vi "PatternMatch_MainFunction.vi"(0 "PatternMatchParameter":T5={"Algorithm"=2, "Match Parameters"={"Number of Matches Requested"=1, "Minimum Match Score"=750.0, "Angle Ranges"=[]}, "ROI Descriptor"={"Global Rectangle"=[], "Contours"=[]}, "Advanced Options"=[{"Item"=1, "Value"=1.0}, {"Item"=103, "Value"=1.0}], "Template path"="", "XOffset"=0, "YOffset"=0} {"ROI Descriptor"."Contours"."Type" items=["No Selection", "Point", "Line", "Rectangle", "Oval", "Polygon", "Freehand Region", "Annulus", "Unused2", "Unused3", "Broken Line", "Freehand Line", "Rotated Rectangle"]; "Advanced Options"."Item" items=["LD Sampling - Minimum Constrast"=0, "LD Sampling - Enable Subpixel Accuracy"=1, "LD Sampling - Search Strategy"=2, "LD Sampling - Subpixel Iterations"=3, "LD Sampling - Subpixel Tolerance"=4, "LD Sampling - Initial Match List Length"=5, "LD Sampling - Match List Reduction Factor"=6, "LD Sampling - Initial Step Size"=7, "LD Sampling - Intermediate Angular Accuracy"=8, "-"=9, "Pyramid - Max Pyramid Level"=100, "Pyramid - Minimum Contrast"=102, "Pyramid - Enable Subpixel Accuracy"=103, "Pyramid - Subpixel Iterations"=104, "Pyramid - Subpixel Tolerance"=105, "Pyramid - Initial Match List Length"=106, "Pyramid - Match List Reduction Factor"=107, "Pyramid - Intermediate Angular Accuracy"=108, "Pyramid - Process Border Matches"=109, "Pyramid - Min Match Separation Distance"=111, "Pyramid - Min Match Separation Angle"=112, "Pyramid - Max Match Overlap"=113, "Pyramid - Max Cache in MB"=114, "Pyramid - Clear Cache"=115]; "Match Parameters"."Angle Ranges"."End Angle" min=-360 max=360; "Match Parameters"."Angle Ranges"."Start Angle" min=-360 max=360; "Match Parameters"."Minimum Match Score" min=0 max=1000; "Match Parameters"."Number of Matches Requested" min=1 max=9999; "Algorithm" items=["All", "Low Discrepancy Sampling", "Grayscale Value Pyramid", "Gradients Pyramid"]}, 5 "Vision_Image In":T1, 9 "ROI Descriptor":T2 {"Contours"."Type" items=["No Selection", "Point", "Line", "Rectangle", "Oval", "Polygon", "Freehand Region", "Annulus", "Unused2", "Unused3", "Broken Line", "Freehand Line", "Rotated Rectangle"]}, 11 "error in":errorcluster) -> (4 "Matches":T4[](array[typedef]) {"Bounding Box"."y" format="%.2g"; "Bounding Box"."x" format="%.2g"; "Score" format="%.2f"; "Scale" format="%.2g"; "Angle" format="%.2g"; "Position"."y" format="%.2g"; "Position"."x" format="%.2g"}, 6 "Matches (real-world)":T3(array[cluster]) {"Bounding Box"."y" format="%.2f"; "Bounding Box"."x" format="%.2f"; "Score" format="%.2f"; "Scale" format="%.2f"; "Angle" format="%.2f"; "Position"."y" format="%.2f"; "Position"."x" format="%.2f"}, 8 "Image (duplicate)":T1(plugin-control), 10 "Number of Matches":i32, 15 "error out":errorcluster)   [LabVIEW 2019]
uses:
  Controls/Parttern Match/Analysis_PatternMatch_Parameter.ctl
  <vilib>/vision/Image Controls.llb/IMAQ Image.ctl
  Controls/Parttern Match/Analysis_PatternMatch_Result.ctl
  <vilib>/vision/NI_Vision_Development_Module.lvlib
panel:
  out "Image":T1(plugin-control)
  out "Template In":T1
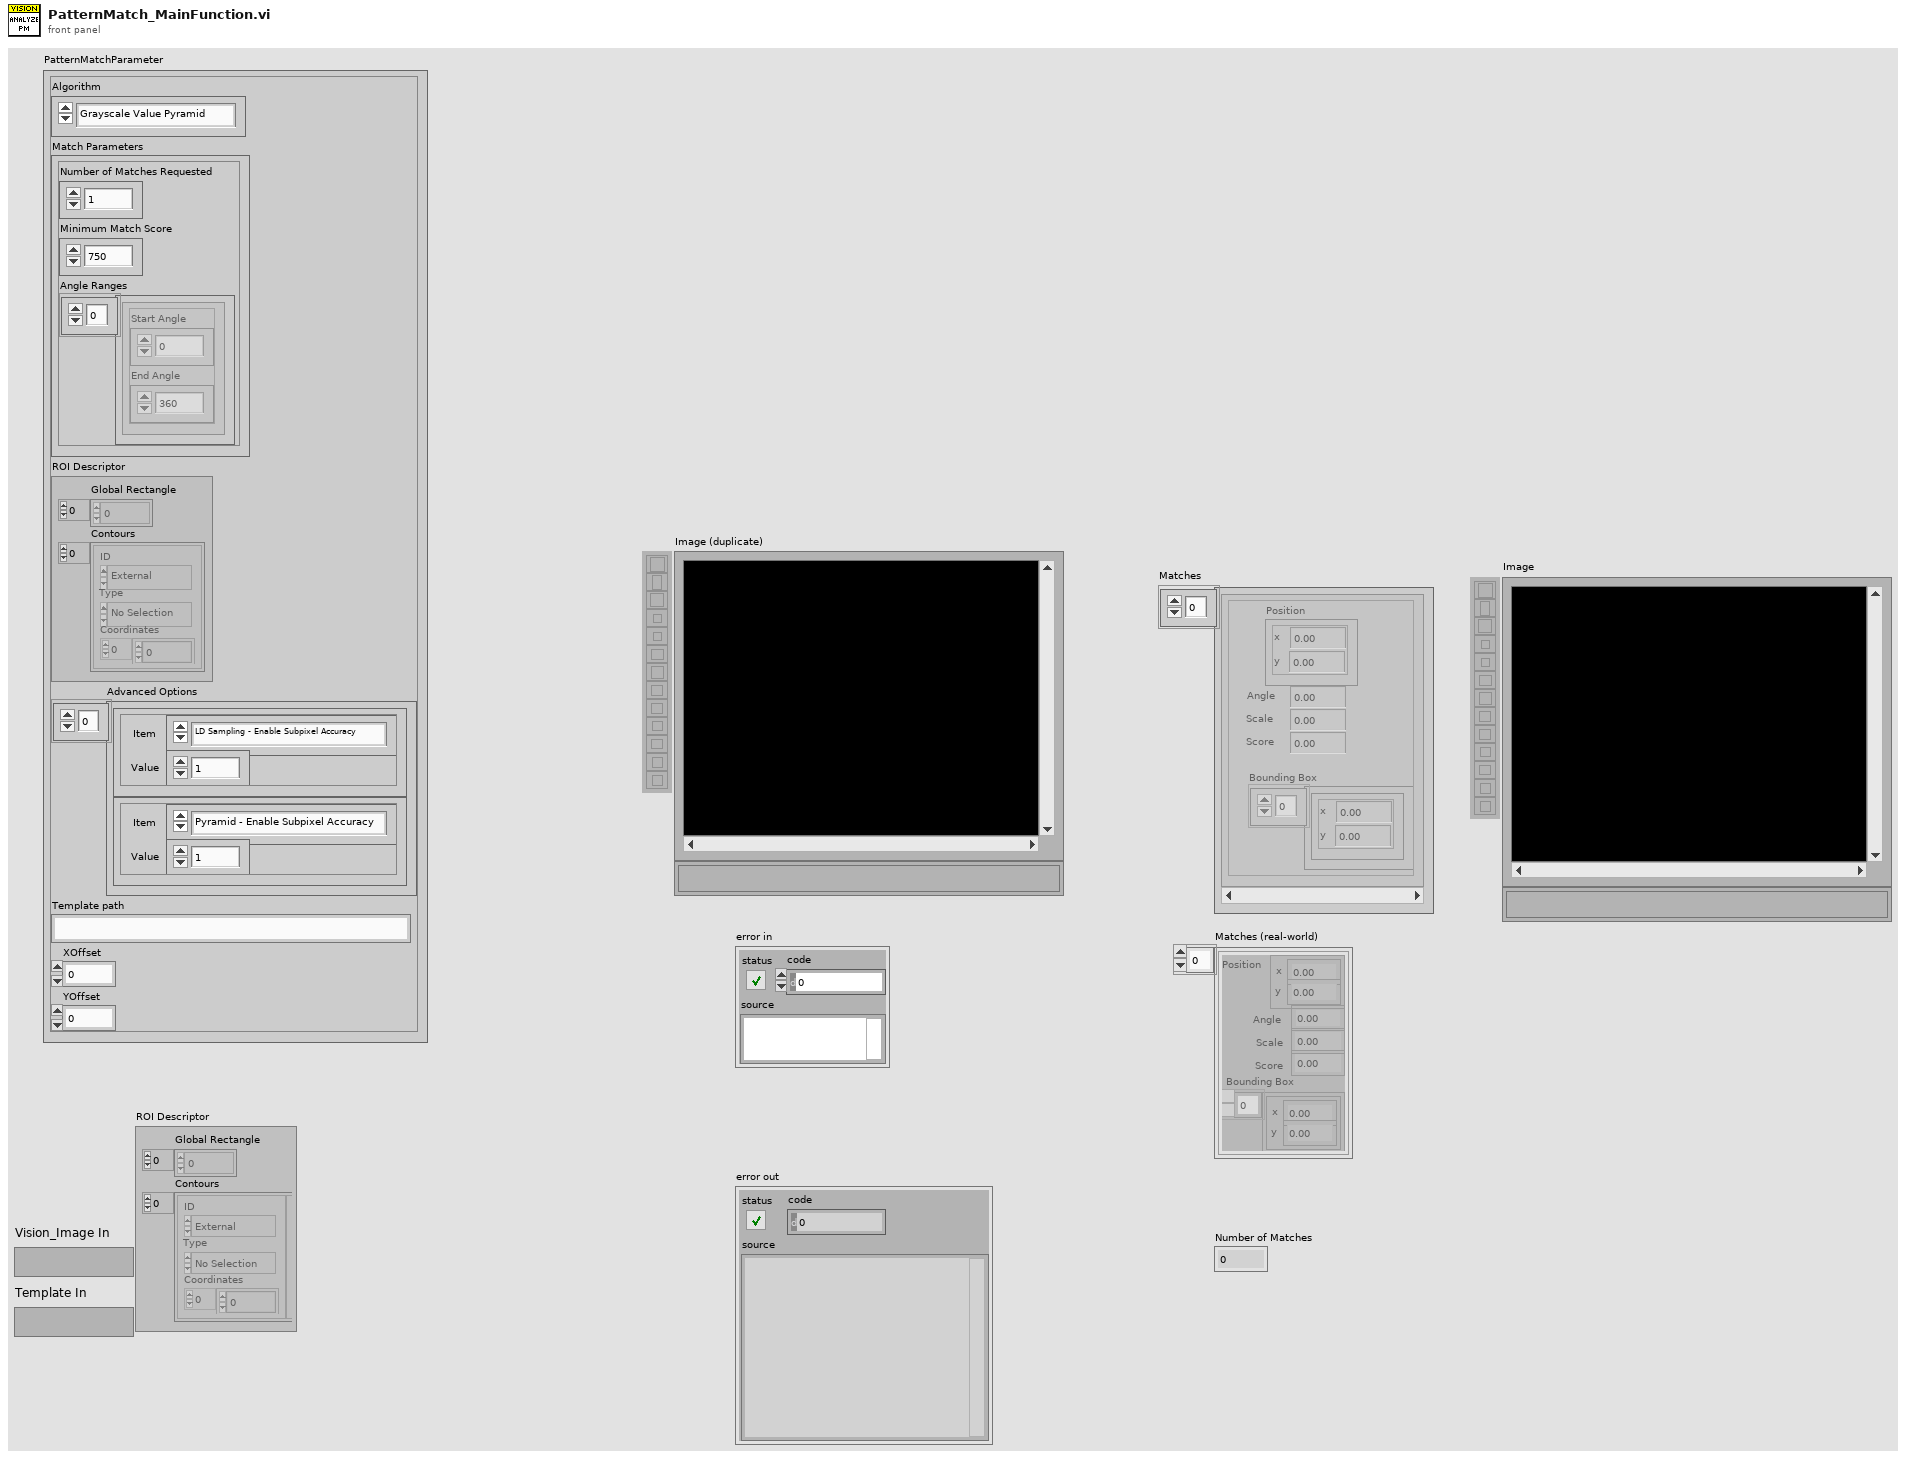
[diagram p1: front panel]
types:
  T1 = typedef "IMAQ Image.ctl" = refnum<image>
  T2 = typedef "ROI Descriptor" = cluster{"Global Rectangle":i32[], "Contours":cluster{"ID":enum32{"External", "Internal"}, "Type":u32, "Coordinates":i32[]}[]}
  T3 = cluster{"Position":cluster{"x":sgl, "y":sgl}, "Angle":sgl, "Scale":sgl, "Score":sgl, "Bounding Box":cluster{"x":sgl, "y":sgl}[]}[]
  T4 = typedef "Analysis_PatternMatch_Result.ctl" = cluster{"Position":cluster{"x":sgl, "y":sgl}, "Angle":sgl, "Scale":sgl, "Score":sgl, "Bounding Box":cluster{"x":sgl, "y":sgl}[]}
  T5 = typedef "Analysis_PatternMatch_Parameter.ctl" = cluster{"Algorithm":i32, "Match Parameters":cluster{"Number of Matches Requested":i32, "Minimum Match Score":sgl, "Angle Ranges":cluster{"Start Angle":sgl, "End Angle":sgl}[]}, "ROI Descriptor":T2, "Advanced Options":cluster{"Item":u16, "Value":dbl}[], "Template path":string, "XOffset":i32, "YOffset":i32}
  T6 = cluster{"Number of Matches Requested":i32, "Minimum Match Score":sgl, "Angle Ranges":cluster{"Start Angle":sgl, "End Angle":sgl}[]}
  T7 = cluster{"Position":cluster{"x":sgl, "y":sgl}, "Angle":sgl, "Scale":sgl, "Score":sgl, "Bounding Box":cluster{"x":sgl, "y":sgl}[]}
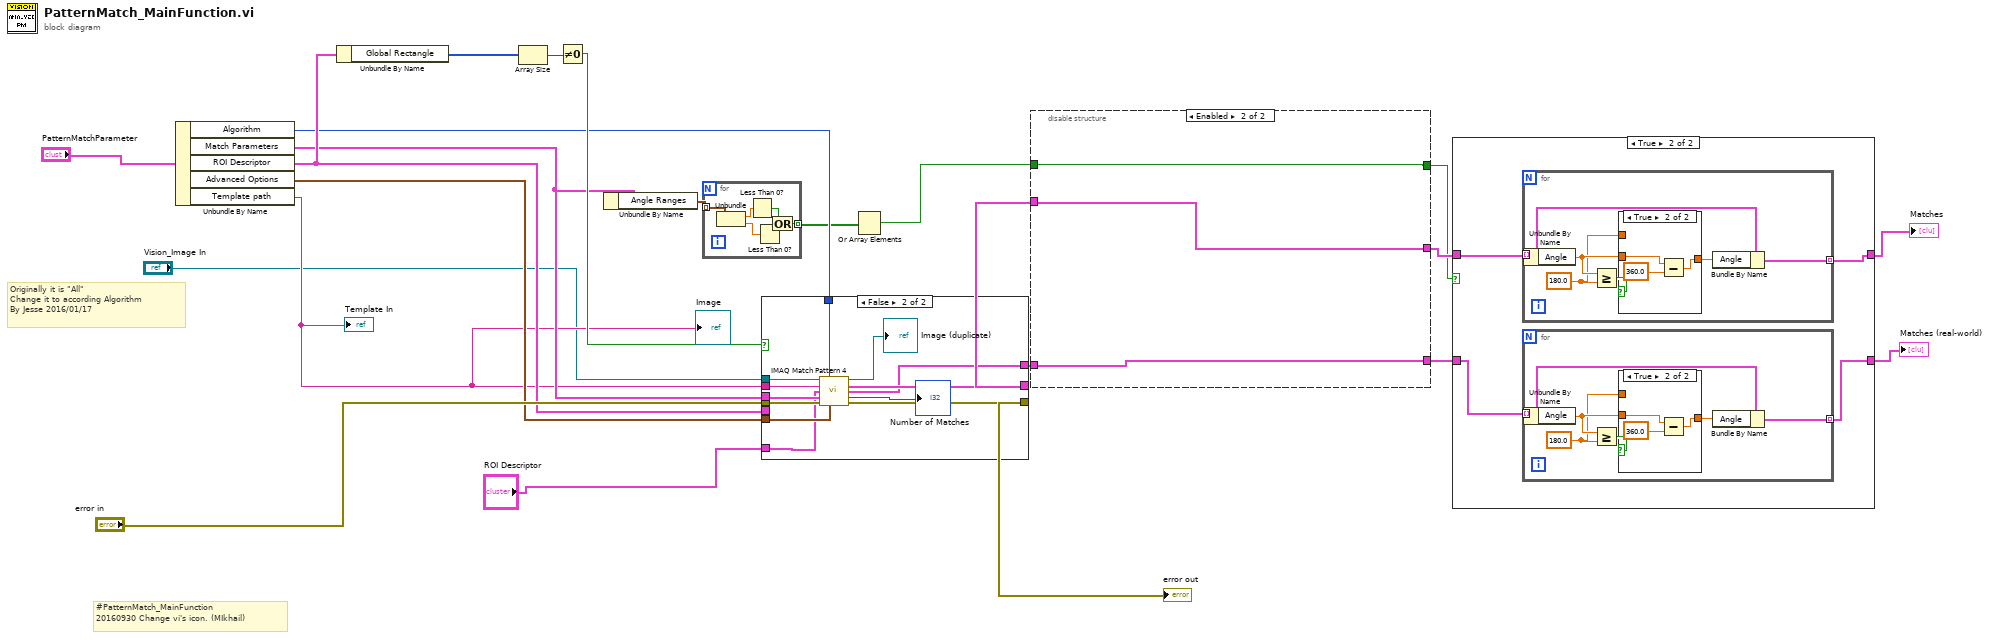
[diagram p0: block diagram]
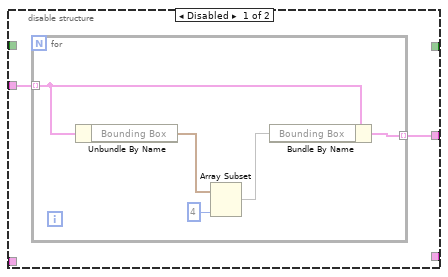
[diagram p5: hidden frame]
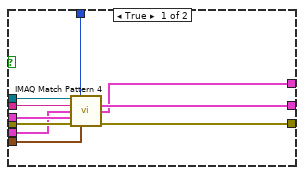
[diagram p6: hidden frame]
diagram:
  # "#PatternMatch_MainFunction\n20160930 Change vi's icon. (MIkhail)"
  # "Originally it is \"All\"\nChange it to according Algorithm\nBy Jesse 2016/01/17"
  n1 = Unbundle By Name("PatternMatchParameter") -> ("Algorithm"=w14:i32, "Match Parameters"=w12:T6, "ROI Descriptor"=w15:T2, "Advanced Options"=w19:cluster{"Item":u16, "Value":dbl}[], "Template path"=w3:string)
  "Template In" <- w3
  "Image" <- w3
  n2 = Unbundle By Name(w15) -> ("Global Rectangle"=w17:i32[])
  n3 = Array Size(array=w17) -> (size(s)=w18:i32)
  n4 = Not Equal To 0?(x=w18) -> (x != 0?=w16:bool)
  n5 = Unbundle By Name(w12) -> ("Angle Ranges"=w4:cluster{"Start Angle":sgl, "End Angle":sgl}[])
  n6 = for {
    tunnel: w4 -> [w29] mode=indexing
    tunnel: [w24] -> w11 mode=indexing
    n7 = Unbundle(w29) -> ("Start Angle"=w28:sgl, "End Angle"=w27:sgl)
    n8 = Less Than 0?(x=w28) -> (x < 0?=w26:bool)
    n9 = Less Than 0?(x=w27) -> (x < 0?=w25:bool)
    n10 = Or(x=w26, y=w25) -> (x .or. y?=w24:bool)
  }
  n11 = case shown="False" w16 {
    tunnel: "error in" -> [w39 w51]
    tunnel: w3 -> [w38 w50]
    tunnel: "Vision_Image In" -> [w37 w49]
    tunnel: w14 -> [w36 w48]
    tunnel: w12 -> [w35 w43]
    tunnel: [w34 w47] -> w21
    tunnel: [w33 w46] -> w20
    tunnel: w19 -> [w32 w45]
    tunnel: w15 -> [w31 _]
    tunnel: [w30 w44] -> w13
    tunnel: "ROI Descriptor" -> [_ w41]
    frame True {
      n12 = call "IMAQ Match Pattern 4"("Image"=w37, "Algorithm"=w36, "Template Image"=w38, "ROI Descriptor"=w31, "Parameters"=w35, "error in (no error)"=w39, "Advanced Options"=w32) -> ("Matches (pixel)"=w33:T3, "Matches (real-world)"=w30:T3, "error out"=w34:errorcluster)  [unwired: 4 in, 2 out]
    }
    frame False {
      n13 = call "IMAQ Match Pattern 4"("Image"=w49, "Algorithm"=w48, "Template Image"=w50, "ROI Descriptor"=w41, "Parameters"=w43, "error in (no error)"=w51, "Advanced Options"=w45) -> ("Image (duplicate)"=→"Image (duplicate)":T1, "Matches (pixel)"=w46:T3, "Matches (real-world)"=w44:T3, "Number of Matches"=→"Number of Matches":i32, "error out"=w47:errorcluster)  [unwired: 4 in]
    }
  }
  "error out" <- w21
  n14 = Or Array Elements(Boolean array=w11) -> (logical OR=w5:bool)
  n15 = disable-structure shown="Enabled" {
    disable-tunnel: w20 -> [w53 w61]
    disable-tunnel: [w52 w61] -> w9
    disable-tunnel: w13 -> [_ w60]
    disable-tunnel: [_ w60] -> w7
    disable-tunnel: [_ w59] -> w6
    disable-tunnel: w5 -> [_ w59]
    frame Disabled {
      n16 = for {
        tunnel: w53 -> [w57] mode=indexing
        tunnel: [w54] -> w52 mode=indexing
        n17 = Unbundle By Name(w57) -> ("Bounding Box"=w56:cluster{"x":sgl, "y":sgl}[])
        n18 = Array Subset(array=w56, length=4) -> (w55:cluster{"x":sgl, "y":sgl}[])  [unwired: 1 in]
        n19 = Bundle By Name(cluster=w57, "Bounding Box"=w55) -> (w54:T7)
      }
    }
    frame Enabled {
    }
  }
  n20 = case shown="True" w6 {
    tunnel: [w63 w66] -> w10
    tunnel: w9 -> [w63 w67]
    tunnel: [w62 w64] -> w8
    tunnel: w7 -> [w62 w65]
    frame False {
    }
    frame True {
      n21 = for {
        tunnel: w67 -> [w80] mode=indexing
        tunnel: [w78] -> w66 mode=indexing
        w81 = sgl 180.0 ("y")
        n22 = Unbundle By Name(w80) -> ("Angle"=w82:sgl)
        n23 = Greater Or Equal?(x=w82, y=w81) -> (x >= y?=w83:bool)
        n24 = case shown="True" w83 {
          tunnel: w82 -> [w84 w86]
          tunnel: w81 -> [_ _]
          tunnel: [w84 w87] -> w79
          frame False {
          }
          frame True {
            n25 = Subtract(x=w86, y=sgl 360.0) -> (x-y=w87:sgl)
          }
        }
        n26 = Bundle By Name(cluster=w80, "Angle"=w79) -> (w78:T7)
      }
      n27 = for {
        tunnel: w65 -> [w70] mode=indexing
        tunnel: [w68] -> w64 mode=indexing
        w71 = sgl 180.0 ("y")
        n28 = Unbundle By Name(w70) -> ("Angle"=w72:sgl)
        n29 = Greater Or Equal?(x=w72, y=w71) -> (x >= y?=w73:bool)
        n30 = case shown="True" w73 {
          tunnel: w72 -> [w74 w76]
          tunnel: w71 -> [_ _]
          tunnel: [w74 w77] -> w69
          frame False {
          }
          frame True {
            n31 = Subtract(x=w76, y=sgl 360.0) -> (x-y=w77:sgl)
          }
        }
        n32 = Bundle By Name(cluster=w70, "Angle"=w69) -> (w68:T7)
      }
    }
  }
  "Matches" <- w10
  "Matches (real-world)" <- w8
